vi "Release SAL.vi"(8 "error in (no error)":errorcluster, 11 "Boot Loader in":refnum<class "Boot Loader.lvclass">) -> (0 "error out":errorcluster, 3 "Boot Loader out":refnum<class "Boot Loader.lvclass">)   [LabVIEW 2016, in "Boot Loader.lvclass"]
uses:
  Boot Loader.lvclass
  SALLV_m1m3/SALLV_m1m3.lvlib
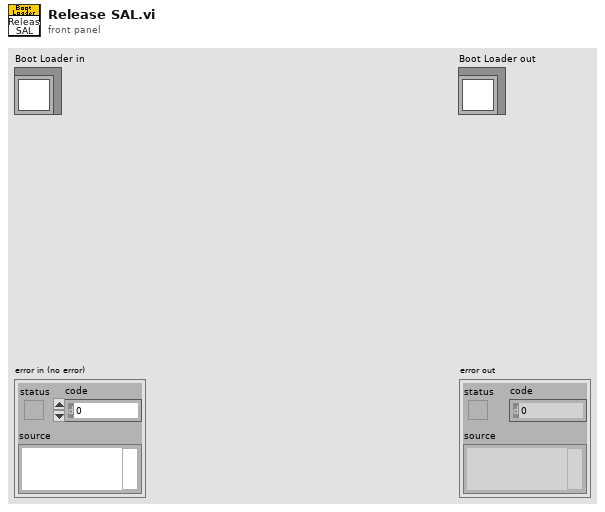
[diagram p1: front panel]
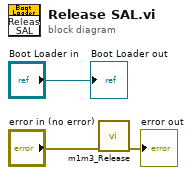
[diagram p0: block diagram]
diagram:
  n1 = call "m1m3_Release.vi"("error in (no error)"="error in (no error)") -> ("error out"=→"error out":errorcluster)  [unwired: 9 in, 1 out]
  "Boot Loader out" <- "Boot Loader in"
